vi "Assert Attach Failed.vi"(8 "error in":errorcluster) -> (0 "error out":errorcluster, 2 "result":string, 3 "pass?":bool)   [LabVIEW 2020, in "MeasurementServerTests.lvlib"]
uses:
  MeasurementServerTests.lvlib
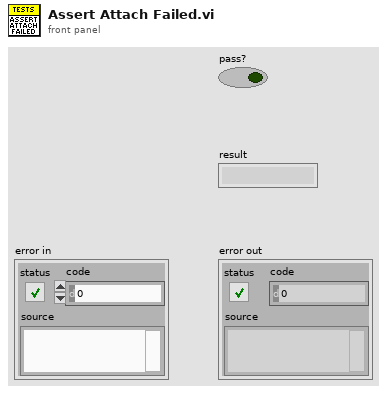
[diagram p1: front panel]
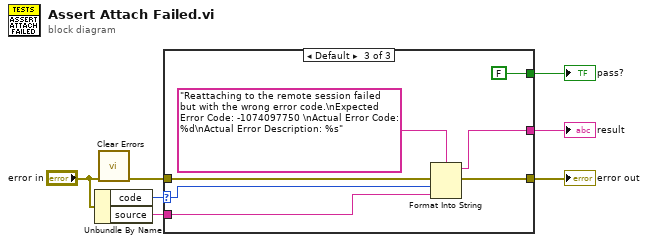
[diagram p0: block diagram]
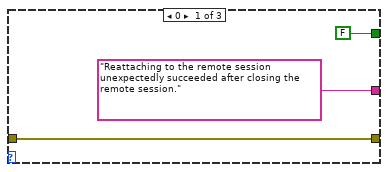
[diagram p2: hidden frame]
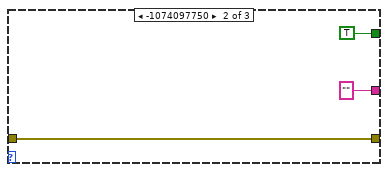
[diagram p3: hidden frame]
diagram:
  n1 = Unbundle By Name("error in") -> ("code"=w3:i32, "source"=w1:string)
  n2 = call <vilib>:"Clear Errors.vi"("error in (no error)"="error in") -> ("error out"=w5:errorcluster)  [unwired: 5 in, 1 out]
  n3 = case shown="Default" w3 {
    selector: w3 -> [_ _ w19]
    tunnel: ["Reattaching to the remote session unexpectedly succeeded after closing the remote session." ("f") "" ("f") w18] -> w7
    tunnel: [FALSE TRUE FALSE] -> w2
    tunnel: w5 -> [w8 w11 w16]
    tunnel: [w8 w11 w15] -> w6
    tunnel: w1 -> [_ _ w14]
    frame 0 {
    }
    frame -1074097750 {
    }
    frame Default {
      n4 = Format Into String(format string="Reattaching to the remote session failed but with the wrong error code.\nExpected Error Code: -1074097750 \nActual Error Code: %d\nActual Error Description: %s" ("f"), error in=w16, w19, w14) -> (resulting string=w18:string, error out=w15:errorcluster)  [unwired: 1 in]
    }
  }
  "result" <- w7
  "error out" <- w6
  "pass?" <- w2
